vi "intial multiple psu test.vi"() -> ()   [LabVIEW 2019]
panel:
  out "Current Einzel Voltage":dbl
  in  "Kd 2":dbl
  in  "Ki 2":dbl
  in  "Kp 2":dbl
  in  "Einzel voltage":dbl(slide) min=0.0 max=3000.0 step=0.183 scale=3.0..3000.0 scale format="%#_7f"
  in  "Einzel Enable":bool
  out "NI 9263(2)":dbl
  in  "?":bool
  out "Current Anode Voltage":dbl
  in  "ANODE VOLTAGE":dbl(slide) min=0.0 max=3000.0 step=0.183 scale=3.0..3000.0 scale format="%#_7f"
  in  "Anode Enable":bool
  out "NI 9263":dbl
  in  "Ki":dbl
  in  "Kd":dbl
  in  "Kp":dbl
  # "at Anode"
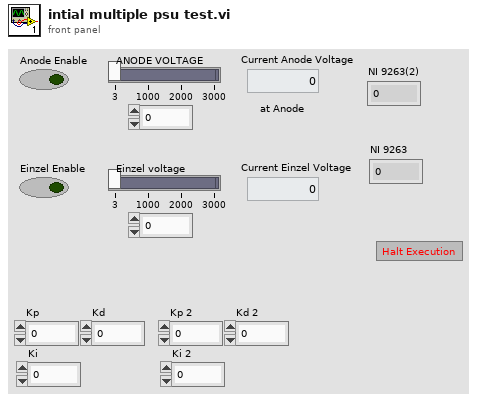
[diagram p1: front panel]
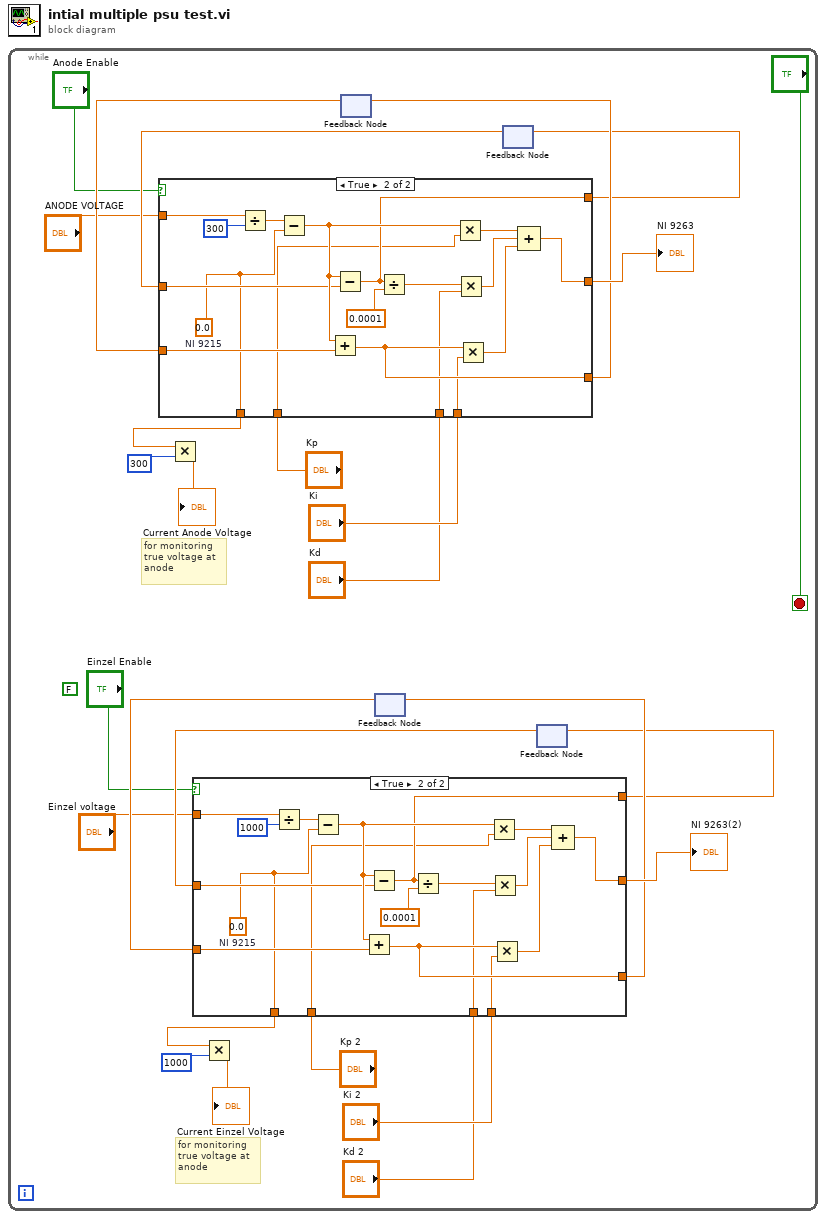
[diagram p0: block diagram]
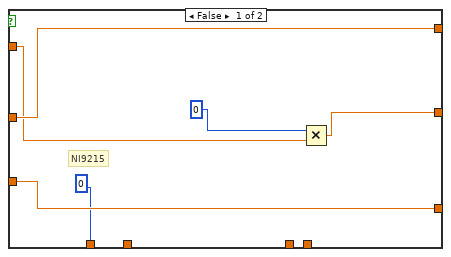
[diagram p2: hidden frame]
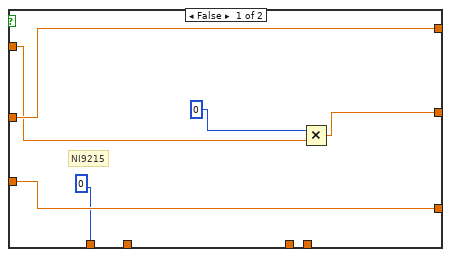
[diagram p3: hidden frame]
diagram:
  n1 = while {
    stop <- "?" stop-if-true
    (unwired) FALSE ("Einzel Enable")
    # "for monitoring \ntrue voltage at\nanode"
    # "for monitoring \ntrue voltage at\nanode"
    n2 = feedback #1() -> (w26:dbl)  [unwired: 1 in]
    n3 = feedback #2() -> (w12:dbl)  [unwired: 1 in]
    n4 = feedback #3() -> (w27:dbl)  [unwired: 1 in]
    n5 = case shown="True" "Anode Enable" {
      tunnel: w27 -> [w57 w67]
      tunnel: [w57 w66] -> w16
      tunnel: w26 -> [w56 w65]
      tunnel: [w56 w64] -> w21
      tunnel: "ANODE VOLTAGE" -> [w54 w63]
      tunnel: [w53 w62] -> w24
      tunnel: "Kp" -> [_ w61]
      tunnel: "Ki" -> [_ w60]
      tunnel: "Kd" -> [_ w59]
      tunnel: [0 w58] -> w17
      frame False {
        # "NI9215"
        n6 = Multiply(x=0, y=w54) -> (x*y=w53:dbl)
      }
      frame True {
        w58 = 0.0  # NI 9215
        n7 = Divide(x=w63, y=300) -> (x/y=w69:dbl)
        n8 = Subtract(x=w69, y=w58) -> (x-y=w74:dbl)
        n9 = Add(x=w74, y=w65) -> (x+y=w64:dbl)
        n10 = Subtract(x=w74, y=w67) -> (x-y=w66:dbl)
        n11 = Divide(x=w66, y=0.0001) -> (x/y=w71:dbl)
        n12 = Multiply(x=w74, y=w61) -> (x*y=w72:dbl)
        n13 = Multiply(x=w71, y=w59) -> (x*y=w68:dbl)
        n14 = Multiply(x=w64, y=w60) -> (x*y=w73:dbl)
        n15 = Compound Arithmetic op=ADD(w72, w68, w73) -> (w62:dbl)
      }
    }
    "NI 9263" <- w24
    n16 = Multiply(x=w17, y=300) -> (x*y=→"Current Anode Voltage":dbl)
    n17 = feedback-in #1(w21) -> ()
    n18 = feedback-in #3(w16) -> ()
    n19 = feedback #4() -> (w13:dbl)  [unwired: 1 in]
    n20 = case shown="True" "Einzel Enable" {
      tunnel: w13 -> [w33 w43]
      tunnel: [w33 w42] -> w2
      tunnel: w12 -> [w32 w41]
      tunnel: [w32 w40] -> w7
      tunnel: "Einzel voltage" -> [w30 w39]
      tunnel: [w29 w38] -> w10
      tunnel: "Kp 2" -> [_ w37]
      tunnel: "Ki 2" -> [_ w36]
      tunnel: "Kd 2" -> [_ w35]
      tunnel: [0 w34] -> w3
      frame False {
        # "NI9215"
        n21 = Multiply(x=0, y=w30) -> (x*y=w29:dbl)
      }
      frame True {
        w34 = 0.0  # NI 9215
        n22 = Divide(x=w39, y=1000) -> (x/y=w45:dbl)
        n23 = Subtract(x=w45, y=w34) -> (x-y=w50:dbl)
        n24 = Add(x=w50, y=w41) -> (x+y=w40:dbl)
        n25 = Subtract(x=w50, y=w43) -> (x-y=w42:dbl)
        n26 = Divide(x=w42, y=0.0001) -> (x/y=w47:dbl)
        n27 = Multiply(x=w50, y=w37) -> (x*y=w48:dbl)
        n28 = Multiply(x=w47, y=w35) -> (x*y=w44:dbl)
        n29 = Multiply(x=w40, y=w36) -> (x*y=w49:dbl)
        n30 = Compound Arithmetic op=ADD(w48, w44, w49) -> (w38:dbl)
      }
    }
    "NI 9263(2)" <- w10
    n31 = Multiply(x=w3, y=1000) -> (x*y=→"Current Einzel Voltage":dbl)
    n32 = feedback-in #2(w7) -> ()
    n33 = feedback-in #4(w2) -> ()
  }
